vi "read_ref.vi"(2 "error in (no error)":errorcluster, 3 "N":i64) -> (0 "error out":errorcluster, 1 "wd":dbl[](array[numeric]))   [LabVIEW 2021]
uses:
  <vilib>/Utility/file.llb/Read Delimited Spreadsheet (DBL).vi
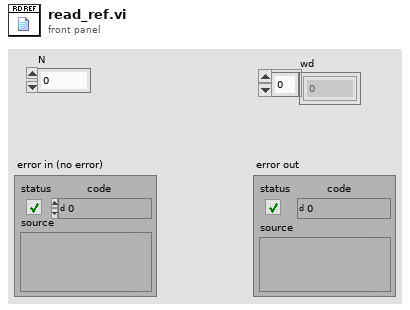
[diagram p1: front panel]
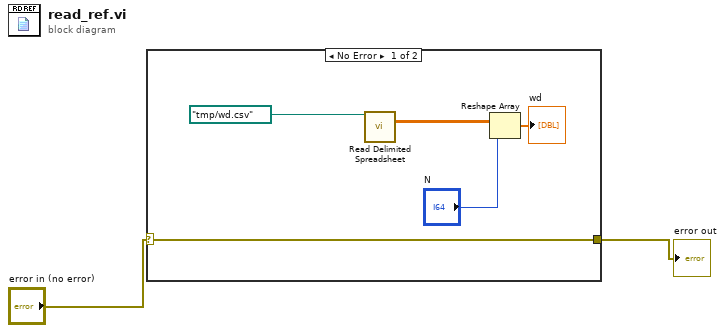
[diagram p0: block diagram]
diagram:
  n1 = case shown="No Error" "error in (no error)" {
    selector: "error in (no error)" -> [w5 w8]
    tunnel: [w5 w8] -> w1
    frame No Error {
      n2 = call-poly <vilib>:"Read Delimited Spreadsheet.vi"("file path (dialog if empty)"=path "/tmp/wd.csv") -> ("all rows"=w7:dbl[][])  [unwired: 9 in, 5 out]
      n3 = Reshape Array(w7, "N") -> (→"wd":dbl[])
    }
    frame Error {
    }
  }
  "error out" <- w1
